vi "ImPro - Insert Image.vi"(8 "error in (no error)":errorcluster, 9 "Rectangle":T1, 10 "24-bit pixmap":u32[][](array[numeric]), 11 "Picture in":refnum<vi>) -> (0 "error out":errorcluster)   [LabVIEW 2023]
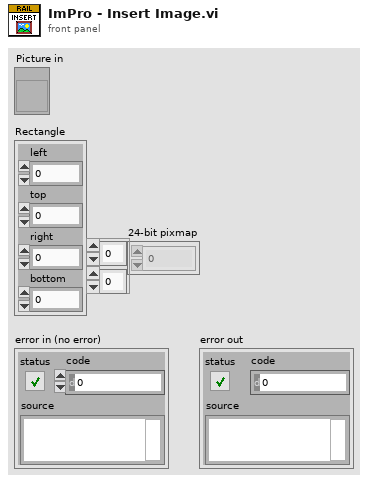
[diagram p1: front panel]
types:
  T1 = cluster{"left":i16, "top":i16, "right":i16, "bottom":i16}
  T2 = typedef "imagedata.ctl" = cluster{"image type":i32, "image depth":i32, "image":u8[], "mask":u8[], "colors":u32[], "Rectangle":cluster{"left":i16, "top":i16, "right":i16, "bottom":i16}}
  T3 = typedef "LVBoundsTypeDef.ctl" = cluster{"Width":u32, "Height":u32}
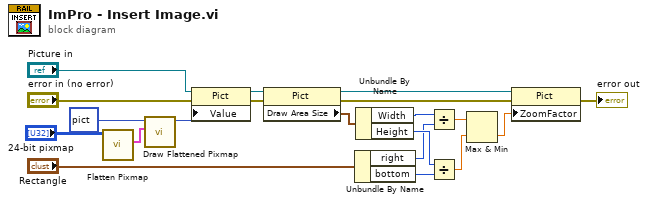
[diagram p0: block diagram]
diagram:
  n1 = call <vilib>:"Flatten Pixmap.vi"("24-bit pixmap"="24-bit pixmap") -> ("image data"=w4:T2)  [unwired: 10 in]
  n2 = call <vilib>:"Draw Flattened Pixmap.vi"("image data"=w4, "picture"=picture data[5B]) -> ("new picture"=w3:picture)  [unwired: 7 in]
  n3 = property class="Pict"(reference="Picture in", error in="error in (no error)", "Value"=w3) -> (reference out=w16:refnum<vi>, error out=w15:errorcluster)
  n4 = property on="Property Node" class="Pict"(reference=w16, error in=w15) -> (reference out=w13:refnum<vi>, error out=w12:errorcluster, "Draw Area Size"=w14:T3)
  n5 = Unbundle By Name("Rectangle") -> ("right"=w6:i16, "bottom"=w5:i16)
  n6 = Unbundle By Name(w14) -> ("Width"=w11:u32, "Height"=w10:u32)
  n7 = Divide(x=w11, y=w6) -> (x/y=w9:dbl)
  n8 = Divide(x=w10, y=w5) -> (x/y=w8:dbl)
  n9 = Max & Min(x=w9, y=w8) -> (min(x,y)=w7:dbl)  [unwired: 1 out]
  n10 = property on="Property Node" class="Pict"(reference=w13, error in=w12, "ZoomFactor"=w7) -> (error out=→"error out":errorcluster)  [unwired: 1 out]
